vi "Is Scaler Type.vi"(3 "Type Enum in":T1) -> (1 "Scaler Type":bool)   [LabVIEW 2013, in "JSONtext.lvlib"]
uses:
  <vilib>/Utility/VariantDataType/Type.ctl
  JSONtext.lvlib
  <vilib>/Utility/VariantDataType/VariantType.lvlib
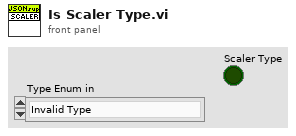
[diagram p1: front panel]
types:
  T1 = typedef "VariantType.lvlib/Type.ctl" = enum8{"Invalid Type", "Void", "I8", "I16", "I32", "I64", "U8", "U16", "U32", "U64", "Single Float", "Double Float", "Extended Float", "Single Complex", "Double Complex", "Extended Complex", "Enum U8", "Enum U16", "Enum U32", "Enum U64", "Single Float With Unit", "Double Float With Unit", "Extended Float With Unit", "Single Complex with Unit", "Double Complex with Unit", "Extended Complex with Unit", "Boolean", "String", "Path", "Picture", "Tag", "Array", "Cluster", "Variant", "LV Variant", "Waveform", "Timestamp", "Digital Waveform", "Digital Data", "ExpressData", "Refnum", "External Data", "VI", "Poly VI", "LabVIEW Class Instance", "Fixed Point"}
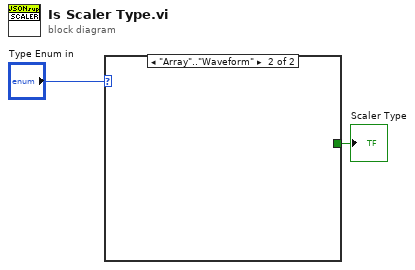
[diagram p0: block diagram]
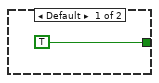
[diagram p2: hidden frame]
diagram:
  n1 = case shown="\"Array\"..\"Waveform\"" "Type Enum in" {
    tunnel: [TRUE _] -> w1
    frame Default {
    }
    frame "Array".."Waveform" {
    }
  }
  "Scaler Type" <- w1
